vi "Set Mathematic Function.vi"(6 "Mathematic function":T1(ring), 8 "error in (no error)":errorcluster, 9 "Mathematical channel (1 to 5)":i32=1, 10 "Channel to process":u16(ring) items=["A1"=0, "A2"=1, "A3"=2, "A4"=3, "A5"=4, "A6"=5, "A7"=6, "A8"=7, "A9"=8, "A10"=9, "K1"=200, "K2"=201, "K3"=202, "K4"=203, "FA1"=204, "FA2"=205, "FA3"=206, "FA4"=207], 11 "VISA resource name":refnum<visa-resource-name>) -> (0 "error out":errorcluster, 3 "VISA resource name out":refnum<visa-resource-name>)   [LabVIEW 2017, in "Sefram DAS220.lvlib"]
doc: "Calculate mathematical function on a channel. Up to 5 mathematical functions. The device screen should be on Graphic F(t) mode to realize calculations."
uses:
  <instrlib>/Sefram DAS220/Sefram DAS220.lvlib
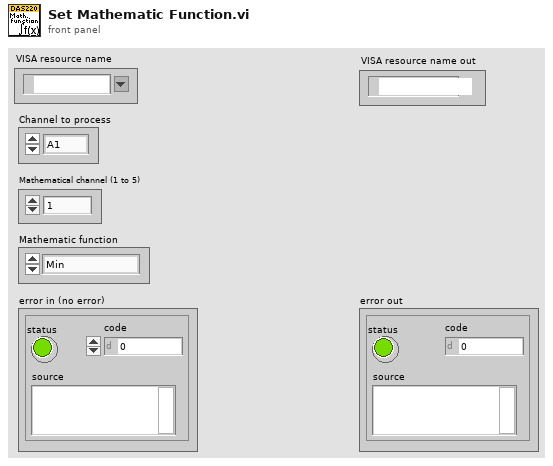
[diagram p1: front panel]
types:
  T1 = enum16{"Min", "Max", "Peak-Peak", "Low Value", "High Value", "Amplitude", "Positive Overshoot", "Negative Overshoot", "Frequency", "Period", "Rising Edge", "Falling Edge", "Positive Width", "Negative Width", "Positive Duty Cycle", "Negative Duty Cycle", "Mean", "RMS", "Standard Deviation"}
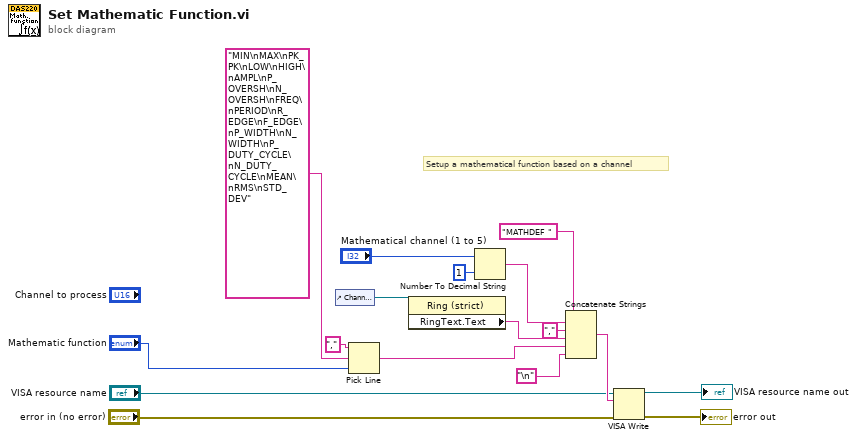
[diagram p0: block diagram]
diagram:
  # "Setup a mathematical function based on a channel"
  n1 = control-ref of="Channel to process"() -> (w1:refnum<vi>)
  n2 = Pick Line(string ("")=",", multi-line string="MIN\nMAX\nPK_PK\nLOW\nHIGH\nAMPL\nP_OVERSH\nN_OVERSH\nFREQ\nPERIOD\nR_EDGE\nF_EDGE\nP_WIDTH\nN_WIDTH\nP_DUTY_CYCLE\nN_DUTY_CYCLE\nMEAN\nRMS\nSTD_DEV", line index="Mathematic function") -> (output string=w10:string)
  n3 = property class="Ring (strict)"(reference=w1) -> ("RingText.Text"=w8:string)  [unwired: 1 in, 2 out]
  n4 = Number To Decimal String(number="Mathematical channel (1 to 5)", width (-)=i16 1) -> (decimal integer string=w4:string)
  n5 = Concatenate Strings("MATHDEF " ("string"), w4, "," ("string"), w8, w10, "\n") -> (w17:string)
  n6 = VISA Write(VISA resource name="VISA resource name", write buffer=w17, error in (no error)="error in (no error)") -> (VISA resource name out=→"VISA resource name out":refnum<visa-resource-name>, error out=→"error out":errorcluster)  [unwired: 1 out]
